vi "ErrorExit.vi"(8 "error in (no error)":errorcluster, 11 "VISA Refnum in":refnum<visa-resource-name>) -> (0 "error out":errorcluster, 3 "VISA Refnum out":refnum<visa-resource-name>)   [LabVIEW 2013]
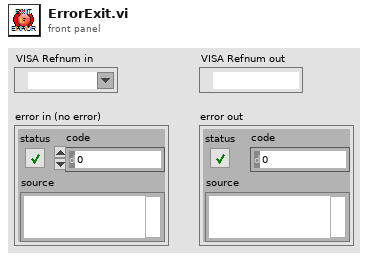
[diagram p1: front panel]
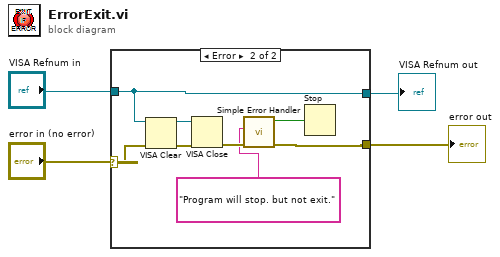
[diagram p0: block diagram]
diagram:
  n1 = case shown="Error" "error in (no error)" {
    selector: "error in (no error)" -> [w6 w8]
    tunnel: [w6 w12] -> w4
    tunnel: "VISA Refnum in" -> [w5 w7]
    tunnel: [w5 w7] -> w3
    frame No Error {
    }
    frame Error {
      n2 = VISA Clear(VISA resource name=w7, error in (no error)=w8) -> (VISA resource name out=w9:refnum<visa-resource-name>, error out=w10:errorcluster)
      n3 = VISA Close(VISA resource name=w9, error in (no error)=w10) -> (error out=w13:errorcluster)
      n4 = call <vilib>:"Simple Error Handler.vi"("error source (\" \")"="Program will stop. but not exit." ("message"), "error in (no error)"=w13) -> ("error?"=w14:bool, "error out"=w12:errorcluster)  [unwired: 3 in, 3 out]
      n5 = Stop(stop? (T)=w14) -> ()
    }
  }
  "error out" <- w4
  "VISA Refnum out" <- w3
